vi "automaticPowerSupplySignal[1].vi"() -> ()   [LabVIEW 2022 SP3]
panel:
  out "FACING RIGHT":bool
  out "REST":bool
  out "FACING LEFT":bool
  in  "PALM ANGLE":dbl
  out "Gyroscope Position":dbl
  in  "MIDDLE FINGER ANGLE":dbl
  out "Finger 2 Position":dbl
  out "Finger 1 Position":dbl
  in  "INDEX FINGER ANGLE":dbl
  in  "stop":bool
  # "PALM POSITION:"
  # "DEGREES"
  # "DEGREES"
  # "DEGREES"
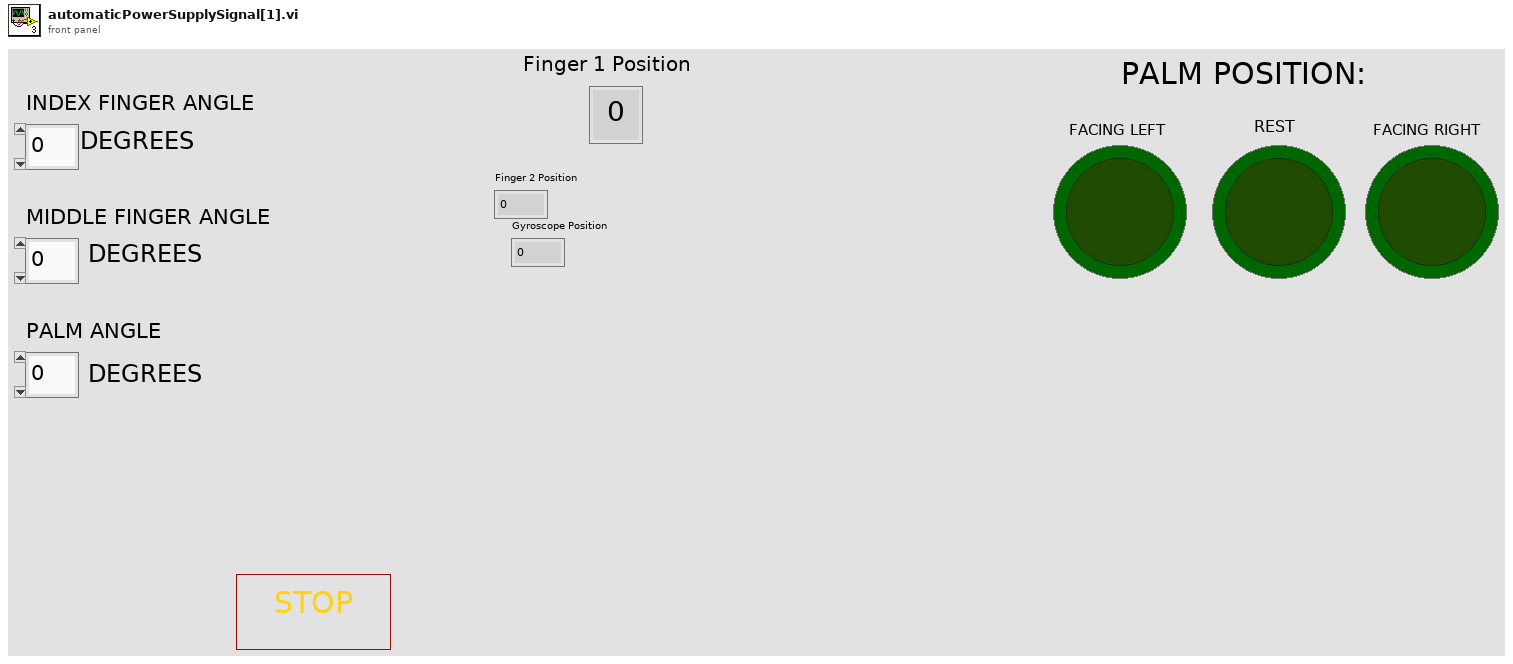
[diagram p1: front panel]
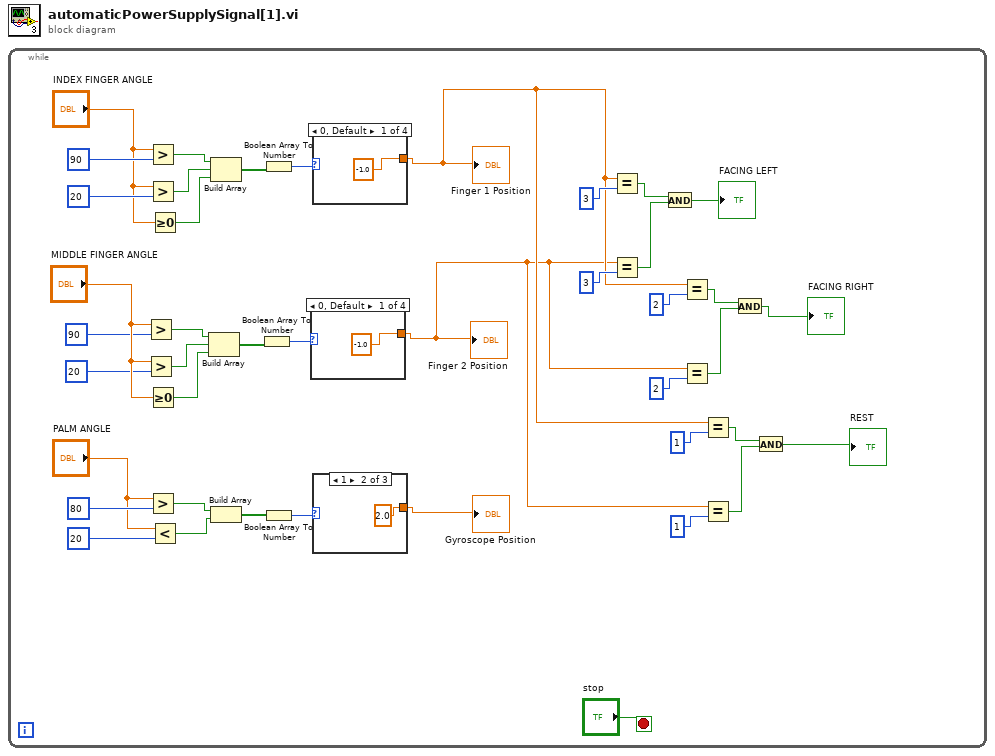
[diagram p0: block diagram]
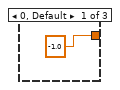
[diagram p2: hidden frame]
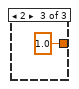
[diagram p3: hidden frame]
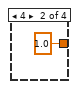
[diagram p4: hidden frame]
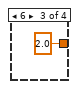
[diagram p5: hidden frame]
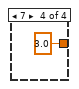
[diagram p6: hidden frame]
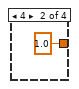
[diagram p7: hidden frame]
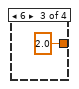
[diagram p8: hidden frame]
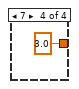
[diagram p9: hidden frame]
diagram:
  n1 = while {
    stop <- "stop" stop-if-true
    n2 = Greater?(x="MIDDLE FINGER ANGLE", y=90) -> (0:w28:bool)
    n3 = Greater?(x="MIDDLE FINGER ANGLE", y=20) -> (0:w29:bool)
    n4 = Greater?(x="INDEX FINGER ANGLE", y=90) -> (0:w39:bool)
    n5 = Greater?(x="INDEX FINGER ANGLE", y=20) -> (0:w38:bool)
    n6 = Greater Or Equal To 0?(x="MIDDLE FINGER ANGLE") -> (x >= 0?=w32:bool)
    n7 = Greater?(x="PALM ANGLE", y=80) -> (0:w24:bool)
    n8 = Greater Or Equal To 0?(x="INDEX FINGER ANGLE") -> (x >= 0?=w35:bool)
    n9 = Less?(x="PALM ANGLE", y=20) -> (x < y?=w19:bool)
    n10 = Build Array(w28, w29, w32) -> (w30:bool[])
    n11 = Build Array(w39, w38, w35) -> (w37:bool[])
    n12 = Build Array(w24, w19) -> (w23:bool[])
    n13 = Boolean Array To Number(Boolean array=w30) -> (number=w31:u32)
    n14 = Boolean Array To Number(Boolean array=w37) -> (number=w36:u32)
    n15 = Boolean Array To Number(Boolean array=w23) -> (number=w18:u32)
    n16 = case shown="0, Default" w31 {
      tunnel: [-1.0 ("Finger 1 Position") 1.0 ("Finger 1 Position") 2.0 ("Finger 1 Position") 3.0 ("Finger 1 Position")] -> w2
      frame 0, Default {
      }
      frame 4 {
      }
      frame 6 {
      }
      frame 7 {
      }
    }
    "Finger 2 Position" <- w2
    n17 = case shown="0, Default" w36 {
      tunnel: [-1.0 ("Finger 1 Position") 1.0 ("Finger 1 Position") 2.0 ("Finger 1 Position") 3.0 ("Finger 1 Position")] -> w3
      frame 0, Default {
      }
      frame 4 {
      }
      frame 6 {
      }
      frame 7 {
      }
    }
    "Finger 1 Position" <- w3
    n18 = case shown="1" w18 {
      tunnel: [-1.0 ("Finger 1 Position") 2.0 ("Finger 1 Position") 1.0 ("Finger 1 Position")] -> w22
      frame 0, Default {
      }
      frame 1 {
      }
      frame 2 {
      }
    }
    "Gyroscope Position" <- w22
    n19 = Equal?(x=w3, y=3) -> (x = y?=w14:bool)
    n20 = Equal?(x=w2, y=3) -> (x = y?=w15:bool)
    n21 = And(x=w14, y=w15) -> (x .and. y?=→"FACING LEFT":bool)
    n22 = Equal?(x=w3, y=2) -> (x = y?=w9:bool)
    n23 = Equal?(x=w2, y=2) -> (x = y?=w10:bool)
    n24 = Equal?(x=w3, y=1) -> (x = y?=w5:bool)
    n25 = Equal?(x=w2, y=1) -> (x = y?=w6:bool)
    n26 = And(x=w9, y=w10) -> (x .and. y?=→"FACING RIGHT":bool)
    n27 = And(x=w5, y=w6) -> (x .and. y?=→"REST":bool)
  }
